vi "AC & DC Estimator.vi"(0 "Signal (V)":dbl[](array[numeric])) -> (1 "AC estimate (Vrms)":dbl format="%0.2f", 2 "DC estimate (V)":dbl format="%0.2f")   [LabVIEW 2017, in "NI_AALPro.lvlib"]
doc: "Estimates the AC and DC levels of the input <B>Signal</B>."
uses:
  NI_AALPro.lvlib
  Hanning Window (DBL).vi
  Mean (DBL).vi
  AllCosWindow (DBL).vi
  NI_AALBase.lvlib
panel:
  # "AC & DC Estimator"
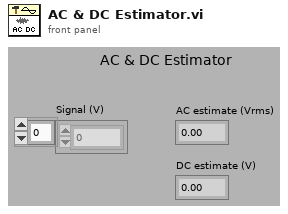
[diagram p1: front panel]
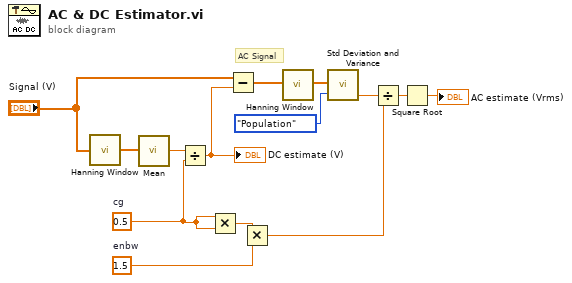
[diagram p0: block diagram]
diagram:
  w7 = 0.5  # cg
  w6 = 1.5  # enbw
  # "AC Signal"
  n1 = call-poly "Hanning Window.vi"("X"="Signal (V)") -> ("Windowed X"=w10:dbl[])  [unwired: 1 out]
  n2 = call-poly "Mean.vi"("X"=w10) -> ("mean"=w8:dbl)  [unwired: 1 out]
  n3 = Divide(x=w8, y=w7) -> (x/y=w9:dbl)
  "DC estimate (V)" <- w9
  n4 = Multiply(x=w7, y=w7) -> (x*y=w5:dbl)
  n5 = Subtract(x="Signal (V)", y=w9) -> (x-y=w3:dbl[])
  n6 = Multiply(x=w5, y=w6) -> (x*y=w4:dbl)
  n7 = call-poly "Hanning Window.vi"("X"=w3) -> ("Windowed X"=w2:dbl[])  [unwired: 1 out]
  n8 = call "Std Deviation and Variance.vi"("X"=w2, "Weighting (Sample)"=enum16{"Sample", "Population"}."Population") -> ("variance"=w12:dbl)  [unwired: 2 out]
  n9 = Divide(x=w12, y=w4) -> (x/y=w14:dbl)
  n10 = Square Root(x=w14) -> (sqrt(x)=→"AC estimate (Vrms)":dbl)
